vi "rethinkdb_msg_sha256.vi"(11 "string":string) -> (3 "sha-256 hash":u32[](array[numeric]) format="%08x")   [LabVIEW 2017]
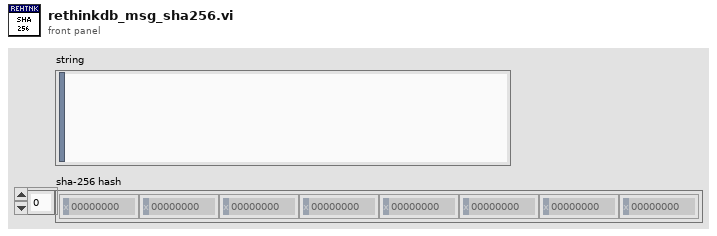
[diagram p1: front panel]
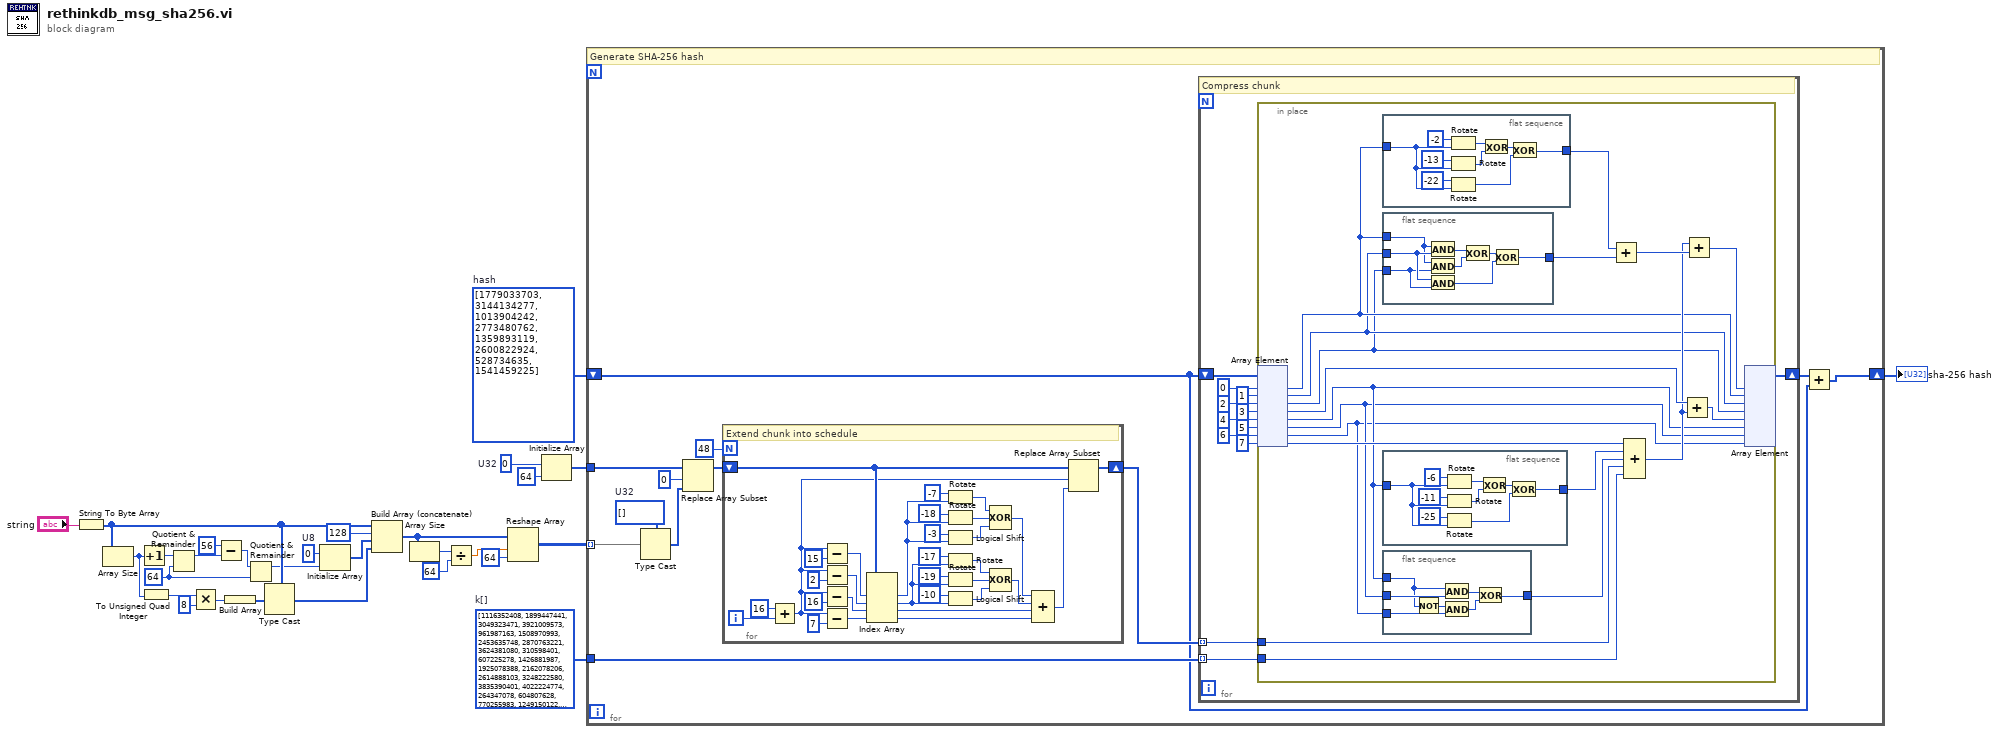
[diagram p0: block diagram]
diagram:
  w18 = u8 0  # U8
  w9 = 64 ("y")
  w23 = u32[] [1116352408, 1899447441, 3049323471, 3921009573, 961987163, 1508970993, 2453635748, 2870763221, 3624381080, 310598401, 607225278, 1426881987, 1925078388, 2162078206, 2614888103, 3248222580, 3835390401, 4022224774, 264347078, 604807628, 770255983, 1249150122, 1555081692, 1996064986, 2554220882, 2821834349, 2952996808, 3210313671, 3336571891, 3584528711, 113926993, 338241895, 666307205, 773529912, 1294757372, 1396182291, 1695183700, 1986661051, 2177026350, 2456956037, 2730485921, 2820302411, 3259730800, 3345764771, 3516065817, 3600352804, 4094571909, 275423344, 430227734, 506948616, 659060556, 883997877, 958139571, 1322822218, 1537002063, 1747873779, 1955562222, 2024104815, 2227730452, 2361852424, 2428436474, 2756734187, 3204031479, 3329325298]  # k[]
  w24 = u32[] [1779033703, 3144134277, 1013904242, 2773480762, 1359893119, 2600822924, 528734635, 1541459225]  # hash
  w27 = u32 0  # U32
  n1 = String To Byte Array(string="string") -> (unsigned byte array=w3:u8[])
  n2 = Array Size(array=w3) -> (size(s)=w8:i32)
  n3 = Increment(x=w8) -> (x+1=w21:i32)
  n4 = To Unsigned Quad Integer(1:w8) -> (0:w7:u64)
  n5 = Quotient & Remainder(x=w21, y=w9) -> (x-y*floor(x/y)=w20:i32)  [unwired: 1 out]
  n6 = Multiply(x=w7, y=u64 8) -> (x*y=w5:u64)
  n7 = Subtract(x=56, y=w20) -> (x-y=w10:i32)
  n8 = Build Array(w5) -> (w4:u64[])
  n9 = Quotient & Remainder(x=w10, y=w9) -> (x-y*floor(x/y)=w1:i32)  [unwired: 1 out]
  n10 = Type Cast(type=w3, x=w4) -> (*(type *) &x=w2:u8[])
  n11 = Initialize Array(w18, w1) -> (w17:u8[])
  n12 = Build Array (concatenate)(w3, u8 128, w17, w2) -> (w13:u8[])
  n13 = Array Size(array=w13) -> (size(s)=w15:i32)
  n14 = Divide(x=w15, y=64) -> (x/y=w12:dbl)
  n15 = Reshape Array(w13, w12, 64 ("dimension size")) -> (w22:u8[][])
  n16 = Initialize Array(w27, 64 ("dimension size")) -> (w25:u32[])
  n17 = for {
    tunnel: w22 -> [w41] mode=indexing
    tunnel: w25 -> [w39]
    tunnel: w23 -> [w34]
    shift-right: [w32] -> w28
    shift-left: w24 -> [w33]
    w40 = u32[] []  # U32
    # "Generate SHA-256 hash"
    n18 = Type Cast(type=w40, x=w41) -> (*(type *) &x=w38:u32[])
    n19 = Replace Array Subset(array=w39, new element=w38, index=0) -> (w36:u32[])
    n20 = for {
      N: 48 -> [_]
      shift-right: [w44] -> w35
      shift-left: w36 -> [w67]
      i -> [w73]
      # "Extend chunk into schedule"
      n21 = Add(x=16, y=w73) -> (x+y=w42:i32)
      n22 = Subtract(x=w42, y=15) -> (x-y=w71:i32)
      n23 = Subtract(x=w42, y=2) -> (x-y=w69:i32)
      n24 = Subtract(x=w42, y=16) -> (x-y=w66:i32)
      n25 = Subtract(x=w42, y=7) -> (x-y=w63:i32)
      n26 = Index Array(array=w67, index #1=w71, index #2=w69, index #3=w66, index #4=w63) -> (element #1=w60:u32, element #2=w53:u32, element #3=w46:u32, element #4=w45:u32)
      n27 = Rotate(1:w60, 2:i16 -7 ("y")) -> (0:w58:u32)
      n28 = Rotate(1:w60, 2:i16 -18 ("y")) -> (0:w57:u32)
      n29 = Logical Shift(y=i16 -3, x=w60) -> (x << y=w56:u32)
      n30 = Rotate(1:w53, 2:i16 -17 ("y")) -> (0:w49:u32)
      n31 = Rotate(1:w53, 2:i16 -19 ("y")) -> (0:w50:u32)
      n32 = Logical Shift(y=i16 -10, x=w53) -> (x << y=w51:u32)
      n33 = Compound Arithmetic op=XOR(w58, w57, w56) -> (w48:u32)
      n34 = Compound Arithmetic op=XOR(w49, w50, w51) -> (w47:u32)
      n35 = Compound Arithmetic op=ADD(w48, w47, w46, w45) -> (w43:u32)
      n36 = Replace Array Subset(array=w67, new element=w43, index=w42) -> (w44:u32[])
    }
    n37 = for {
      tunnel: w35 -> [w76] mode=indexing
      tunnel: w34 -> [w75] mode=indexing
      shift-right: [w74] -> w30
      shift-left: w33 -> [w85]
      # "Compress chunk"
      n38 = in-place {
        in-place-border: w76 -> [w102]
        in-place-border: w75 -> [w101]
        n39 = in-place-array #1(w85, 0, 1, 2, 3, 4, 5, 6, 7) -> (w94:u32, w93:u32, w92:u32, w100:u32, w89:u32, w88:u32, w87:u32, w103:u32)
        n40 = flat-sequence {
          tunnel: w94 -> [w133]
          tunnel: [w128] -> w95
          frame #0 {
            n41 = Rotate(1:w133, 2:i16 -2 ("y")) -> (0:w132:u32)
            n42 = Rotate(1:w133, 2:i16 -13 ("y")) -> (0:w131:u32)
            n43 = Rotate(1:w133, 2:i16 -22 ("y")) -> (0:w129:u32)
            n44 = Exclusive Or(1:w131, 2:w132) -> (0:w130:u32)
            n45 = Exclusive Or(1:w129, 2:w130) -> (0:w128:u32)
          }
        }
        n46 = flat-sequence {
          tunnel: w93 -> [w127]
          tunnel: w92 -> [w126]
          tunnel: w94 -> [w125]
          tunnel: [w120] -> w91
          frame #0 {
            n47 = And(x=w125, y=w127) -> (x .and. y?=w124:u32)
            n48 = And(x=w125, y=w126) -> (x .and. y?=w123:u32)
            n49 = And(x=w127, y=w126) -> (x .and. y?=w121:u32)
            n50 = Exclusive Or(1:w123, 2:w124) -> (0:w122:u32)
            n51 = Exclusive Or(1:w121, 2:w122) -> (0:w120:u32)
          }
        }
        n52 = flat-sequence {
          tunnel: w89 -> [w116]
          tunnel: [w111] -> w90
          frame #0 {
            n53 = Rotate(1:w116, 2:i16 -6 ("y")) -> (0:w115:u32)
            n54 = Rotate(1:w116, 2:i16 -11 ("y")) -> (0:w114:u32)
            n55 = Rotate(1:w116, 2:i16 -25 ("y")) -> (0:w112:u32)
            n56 = Exclusive Or(1:w114, 2:w115) -> (0:w113:u32)
            n57 = Exclusive Or(1:w112, 2:w113) -> (0:w111:u32)
          }
        }
        n58 = flat-sequence {
          tunnel: w88 -> [w110]
          tunnel: w89 -> [w109]
          tunnel: w87 -> [w107]
          tunnel: [w104] -> w86
          frame #0 {
            n59 = Not(x=w109) -> (.not. x?=w108:u32)
            n60 = And(x=w109, y=w110) -> (x .and. y?=w106:u32)
            n61 = And(x=w108, y=w107) -> (x .and. y?=w105:u32)
            n62 = Exclusive Or(1:w105, 2:w106) -> (0:w104:u32)
          }
        }
        n63 = Add(x=w95, y=w91) -> (x+y=w98:u32)
        n64 = Compound Arithmetic op=ADD(w103, w90, w86, w102, w101) -> (w96:u32)
        n65 = Add(x=w100, y=w96) -> (x+y=w99:u32)
        n66 = Add(x=w96, y=w98) -> (x+y=w97:u32)
        n67 = in-place-array #1(w97, w94, w93, w92, w99, w89, w88, w87) -> (w74:u32[])  [unwired: 8 out]
      }
    }
    n68 = Add(x=w30, y=w33) -> (x+y=w32:u32[])
  }
  "sha-256 hash" <- w28
